vi "Remove illegal file characters.vi"(11 "Filename In":string) -> (3 "Filename Out":string)   [LabVIEW 2018]
uses:
  <vilib>/regexp/Match Regular Expression.xnode
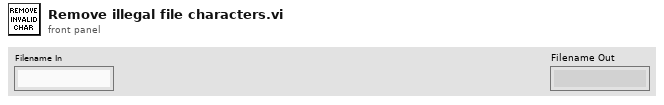
[diagram p1: front panel]
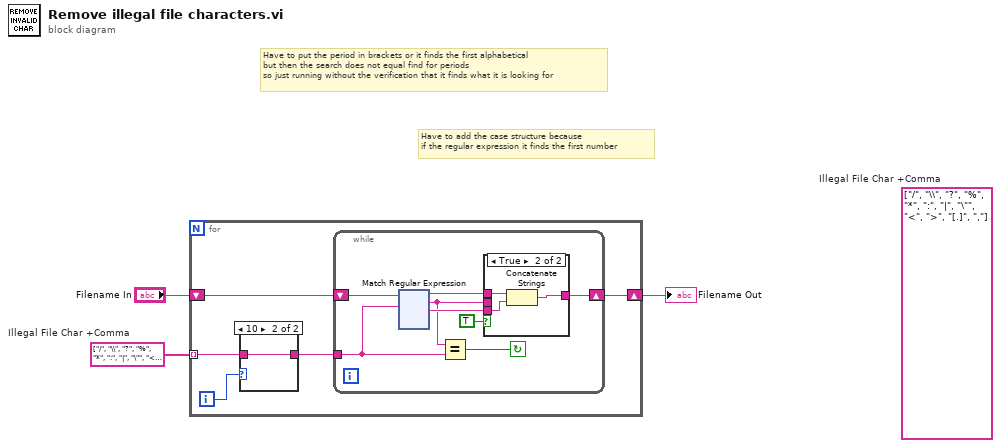
[diagram p0: block diagram]
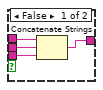
[diagram p3: hidden frame]
diagram:
  (unwired) string[] ["/", "\\", "?", "%", "*", ":", "|", "\"", "<", ">", "[.]", ","]  # Illegal File Char +Comma
  w1 = string[] ["/", "\\", "?", "%", "*", ":", "|", "\"", "<", ">", "[.]", ","]  # Illegal File Char +Comma
  # "Have to put the period in brackets or it finds the first alphabetical\nbut then the search does not equal find for periods\nso just running without the verification that it finds what it is looking for"
  # "Have to add the case structure because\nif the regular expression it finds the first number"
  n1 = for {
    shift-right: [w7] -> w3
    shift-left: "Filename In" -> [w8]
    tunnel: w1 -> [w5] mode=indexing
    i -> [w6]
    n2 = case shown="10" w6 {
      tunnel: w5 -> [w9 w10]
      tunnel: [w9 w10] -> w4
      frame Default {
      }
      frame 10 {
      }
    }
    n3 = while {
      tunnel: w4 -> [w15]
      shift-right: [w12] -> w7
      shift-left: w8 -> [w18]
      stop <- w14 continue-if-true
      n4 = xnode "Match Regular Expression"("input string"=w18, "regular expression"=w15) -> ("before match"=w17:string, "whole match"=w13:string, "after match"=w16:string)  [unwired: 4 in, 2 out]
      n5 = Equal?(x=w13, y=w15) -> (x = y?=w14:bool)
      n6 = case shown="True" TRUE {
        tunnel: w17 -> [w21 w25]
        tunnel: w16 -> [w22 w24]
        tunnel: [w20 w23] -> w12
        tunnel: w13 -> [w19 _]
        frame False {
          n7 = Concatenate Strings(w21, w19, w22) -> (w20:string)
        }
        frame True {
          n8 = Concatenate Strings(w25, w24) -> (w23:string)
        }
      }
    }
  }
  "Filename Out" <- w3
